vi "Set PID.vi"(8 "error in":errorcluster, 10 "PID Params":cluster{"P":sgl, "I":sgl, "D":sgl}, 11 "TE Cooler in":refnum<class "TE Cooler.lvclass">) -> (0 "error out":errorcluster, 3 "TE Cooler out":refnum<class "TE Cooler.lvclass">)   [LabVIEW 2018, in "TE Cooler.lvlib" / "TE Cooler.lvclass"]
doc: "Updates the control parameters (P = proportional, I = integral, D = derivative) in both the object and on the controller itself."
uses:
  TE Cooler.lvclass
  Controls/Command.ctl
  TE Cooler.lvclass/TE Cooler.ctl
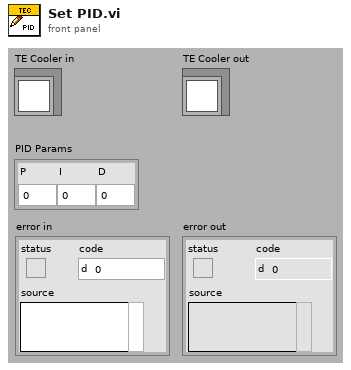
[diagram p1: front panel]
types:
  T1 = typedef "TE Cooler.lvlib/TE Cooler.lvclass/Command.ctl" = enum16{"INPUT1", "DESIRED CONTROL VALUE", "POWER OUTPUT", "ALARM STATUS", "INPUT 2", "OUTPUT CURRENT COUNTS", "ALARM TYPE", "SET TYPE DEFINE", "SENSOR TYPE", "CONTROL TYPE", "CONTROL OUTPUT POLARITY", "POWER ON/OFF", "OUTPUT SHUTDOWN IF ALARM", "FIXED DESIRED CONTROL SETTING", "PROPORTIONAL BANDWIDTH", "INTEGRAL GAIN", "DERIVATIVE GAIN", "LOW EXTERNAL SET RANGE", "HIGH EXTERNAL SET RANGE", "ALARM DEADBAND", "HIGH ALARM SETTING", "LOW ALARM SETTING", "CONTROL DEADBAND SETTING", "INPUT1 OFFSET", "INPUT2 OFFSET", "HEAT MULTIPLIER", "COOL MULTIPLIER", "OVER CURRENT COUNT COMPARE VALUE", "ALARM LATCH ENABLE", "NOT USED", "ALARM LATCH RESET", "CHOOSE SENSOR FOR ALARM FUNCTION", "CHOOSE TEMPERATURE WORKING UNITS", "EEPROM WRITE ENABLE", "OVER CURRENT CONTINUOUS", "OVER CURRENT RESTART ATTEMPTS", "JP3 DISPLAY ENABLE"}
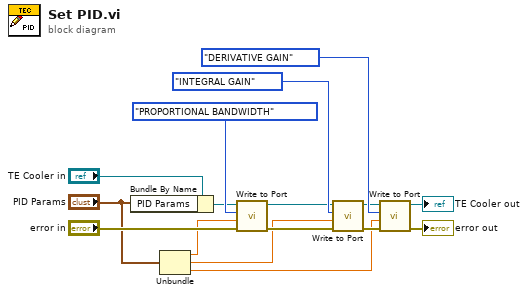
[diagram p0: block diagram]
diagram:
  n1 = Bundle By Name(cluster="TE Cooler in", "PID Params"="PID Params") -> (w4:refnum<class "TE Cooler.lvclass">)
  n2 = Unbundle("PID Params") -> ("P"=w3:sgl, "I"=w2:sgl, "D"=w1:sgl)
  n3 = call "Write to Port.vi"("error in"="error in", "Input Value"=w3, "TEC Cmd"=Command."PROPORTIONAL BANDWIDTH", "TE Cooler in"=w4) -> ("error out"=w6:errorcluster, "TE Cooler out"=w8:refnum<class "TE Cooler.lvclass">)  [unwired: 5 in, 1 out]
  n4 = call "Write to Port.vi"("error in"=w6, "Input Value"=w2, "TEC Cmd"=Command."INTEGRAL GAIN", "TE Cooler in"=w8) -> ("error out"=w5:errorcluster, "TE Cooler out"=w7:refnum<class "TE Cooler.lvclass">)  [unwired: 5 in, 1 out]
  n5 = call "Write to Port.vi"("error in"=w5, "Input Value"=w1, "TEC Cmd"=Command."DERIVATIVE GAIN", "TE Cooler in"=w7) -> ("error out"=→"error out":errorcluster, "TE Cooler out"=→"TE Cooler out":refnum<class "TE Cooler.lvclass">)  [unwired: 5 in, 1 out]
